vi "GetMouse.vi"(8 "error in (no error)":errorcluster, 11 "Input in":refnum<class "Input.lvclass">) -> (0 "error out":errorcluster, 1 "button info":T2, 2 "axis info":T1, 3 "Input out":refnum<class "Input.lvclass">)   [LabVIEW 2009, in "Input.lvclass"]
uses:
  Input.lvclass
  Input.lvclass/Input.ctl
  <vilib>/Utility/inputDevices.llb/mouseAcquire.vi
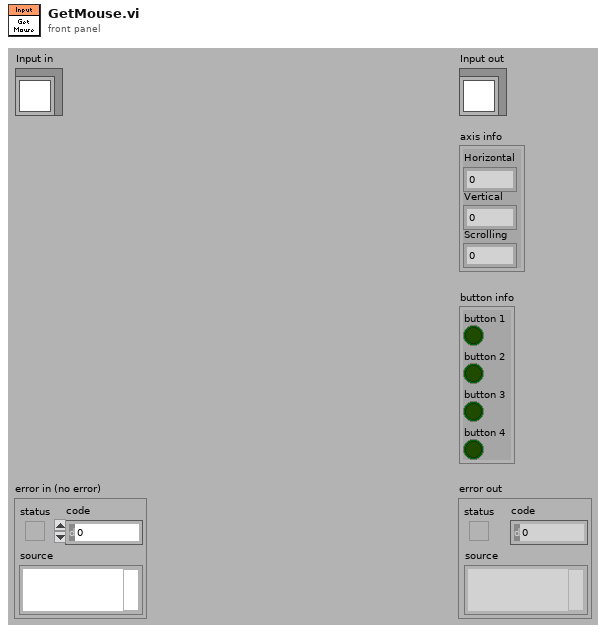
[diagram p1: front panel]
types:
  T1 = cluster{"Horizontal":i32, "Vertical":i32, "Scrolling":i32}
  T2 = cluster{"button 1":bool, "button 2":bool, "button 3":bool, "button 4":bool}
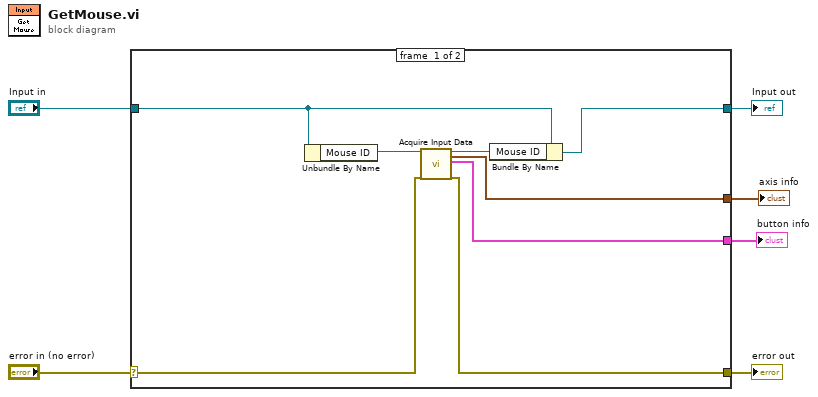
[diagram p0: block diagram]
diagram:
  n1 = case shown="No Error" "error in (no error)" {
    selector: "error in (no error)" -> [w10 w16]
    tunnel: [w9 w16] -> w5
    tunnel: [w12 w15] -> w3
    tunnel: "Input in" -> [w13 w15]
    tunnel: [w8 _] -> w2
    tunnel: [w7 _] -> w1
    frame #0 {
      n2 = Unbundle By Name(w13) -> ("Mouse ID"=w14:refnum<k1>)
      n3 = call-poly <vilib>:"Acquire Input Data.vi"("device ID"=w14, "error in (no error)"=w10) -> ("device ID"=w11:refnum<k1>, "axis info"=w7:T1, "button info"=w8:T2, "error out"=w9:errorcluster)  [unwired: 14 in]
      n4 = Bundle By Name(cluster=w13, "Mouse ID"=w11) -> (w12:refnum<class "Input.lvclass">)
    }
    frame #1 {
    }
  }
  "error out" <- w5
  "Input out" <- w3
  "button info" <- w2
  "axis info" <- w1
